vi "UUIDs - Convert UUID Formula String to LabView.vi"(8 "error in (no error)":errorcluster, 10 "All UUIDs":string[](array[string])=["P1", "Valve", "Temp1", "Press2", "Temp2", "mFlow"], 11 "UUID Fromula String":string="mFlow*1000*(Temp2-Temp1)") -> (0 "error out":errorcluster, 1 "Formula Variables":string[](array[string])=["a0", "a1", "a2"], 2 "Formula UUIDs":string[](array[string])=["Temp1", "Temp2", "mFlow"], 3 "LabView Formula String":string="a2*1000*(a1-a0)")   [LabVIEW 2020]
uses:
  Delete Elements From Array/Delete Elements From Array - string.vi
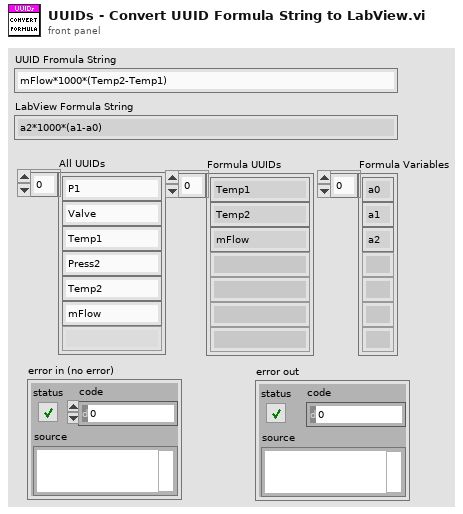
[diagram p1: front panel]
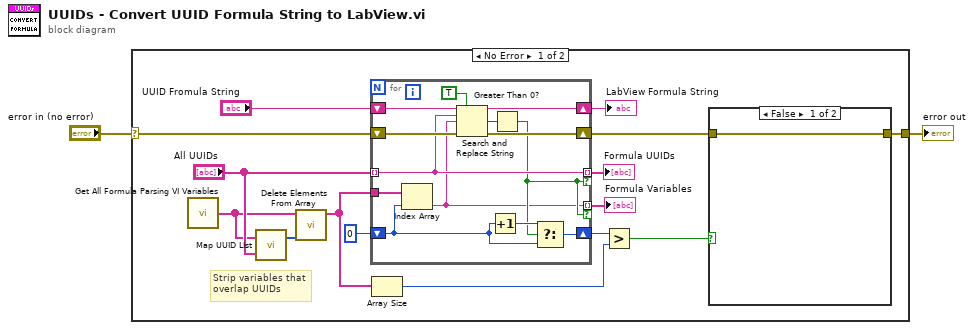
[diagram p0: block diagram]
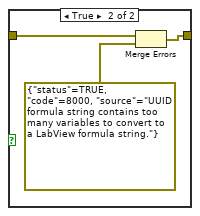
[diagram p2: hidden frame]
diagram:
  n1 = case shown="No Error" "error in (no error)" {
    selector: "error in (no error)" -> [w11 w35]
    tunnel: [w8 w35] -> w2
    frame No Error {
      # "Strip variables that\noverlap UUIDs"
      n2 = call "Get All Formula Parsing VI Variables.vi"() -> ("All Variables"=w3:string[])
      n3 = call "Map UUID LIst.vi"("UUIDs"="All UUIDs", "UUID List"=w3) -> ("indices"=w6:i32[])  [unwired: 1 out]
      n4 = call-poly "Delete Elements From Array.vi"("indices (none)"=w6, "1D Array"=w3) -> ("array w/ subset deleted"=w5:string[])  [unwired: 8 in, 1 out]
      n5 = for {
        shift-right: [w33] -> w15
        shift-left: "UUID Fromula String" -> [w34]
        tunnel: "All UUIDs" -> [w28] mode=indexing
        shift-right: [w31] -> w16
        shift-left: w11 -> [w32]
        shift-right: [w30] -> w10
        shift-left: 0 -> [w24]
        tunnel: w5 -> [w25]
        tunnel: [w28] -> w14 mode=indexing if=w27
        tunnel: [w23] -> w17 mode=indexing if=w27
        n6 = Index Array(array=w25, index=w24) -> (element=w23:string)
        n7 = Search and Replace String(replace all?=TRUE ("replace all? (F)"), input string=w34, search string=w28, replace string=w23, error in=w32) -> (result string=w33:string, number of replacements=w26:i32, error out=w31:errorcluster)  [unwired: 3 in, 1 out]
        n8 = Increment(x=w24) -> (x+1=w29:i32)
        n9 = Greater Than 0?(x=w26) -> (x > 0?=w27:bool)
        n10 = Select(t=w29, s=w27, f=w24) -> (s? t:f=w30:i32)
      }
      "LabView Formula String" <- w15
      "Formula UUIDs" <- w14
      "Formula Variables" <- w17
      n11 = Array Size(array=w5) -> (size(s)=w9:i32)
      n12 = Greater?(x=w10, y=w9) -> (0:w7:bool)
      n13 = case shown="False" w7 {
        tunnel: w16 -> [w18 w21]
        tunnel: [w18 w20] -> w8
        frame False {
        }
        frame True {
          n14 = Merge Errors(w21, errorcluster {"status"=TRUE, "code"=8000, "source"="UUID formula string contains too many variables to convert to a LabView formula string."} ("error in")) -> (w20:errorcluster)
        }
      }
    }
    frame Error {
    }
  }
  "error out" <- w2
